vi "Get Cluster Info of Variant.vi"(8 "error in (no error)":errorcluster, 11 "Cluster Variant":variant) -> (0 "error out":errorcluster, 1 "mem_size":i32, 2 "byte_alignment":i16, 3 "Cluster Info":T1[](array[typedef]), 4 "flattstring_size":u32)   [LabVIEW 2021, in "DataTypes_CIF_U.lvlib"]
uses:
  DataTypes_CIF_U.lvlib
  Typedef/Cluster Info.ctl
  <vilib>/Utility/Data Type/Type Definitions/Data Type.ctl
  Typedef/Errors.ctl
  Errors/Append Error Location.vi
  <vilib>/Utility/Data Type/NI_Data Type.lvlib
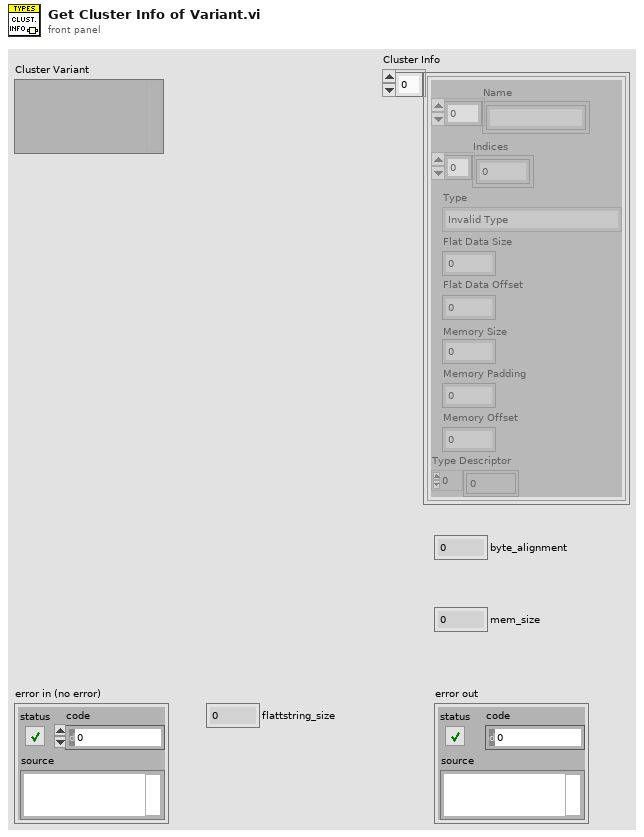
[diagram p1: front panel]
types:
  T1 = typedef "DataTypes_CIF_U.lvlib/Cluster Info.ctl" = cluster{"Name":string[], "Indices":i32[], "Type":T2, "Flat Data Size":u32, "Flat Data Offset":u32, "Memory Size":u32, "Memory Padding":u32, "Memory Offset":u32, "Type Descriptor":i16[]}
  T2 = typedef "NI_Data Type.lvlib/Data Type.ctl" = enum8{"Invalid Type", "Void", "I8", "I16", "I32", "I64", "U8", "U16", "U32", "U64", "Single Float", "Double Float", "Extended Float", "Single Complex", "Double Complex", "Extended Complex", "Enum U8", "Enum U16", "Enum U32", "Enum U64", "Single Float With Unit", "Double Float With Unit", "Extended Float With Unit", "Single Complex with Unit", "Double Complex with Unit", "Extended Complex with Unit", "Boolean", "String", "Path", "Picture", "Tag", "Array", "Cluster", "Variant", "LV Variant", "Waveform", "Timestamp", "Digital Waveform", "Digital Data", "ExpressData", "Refnum", "External Data", "VI", "Poly VI", "LabVIEW Class Instance", "Fixed Point", "Set Collection", "Map Collection"}
  T3 = typedef "DataTypes_CIF_U.lvlib/Errors.ctl" = enum16{"Too few bytes", "Unsupported Type"}
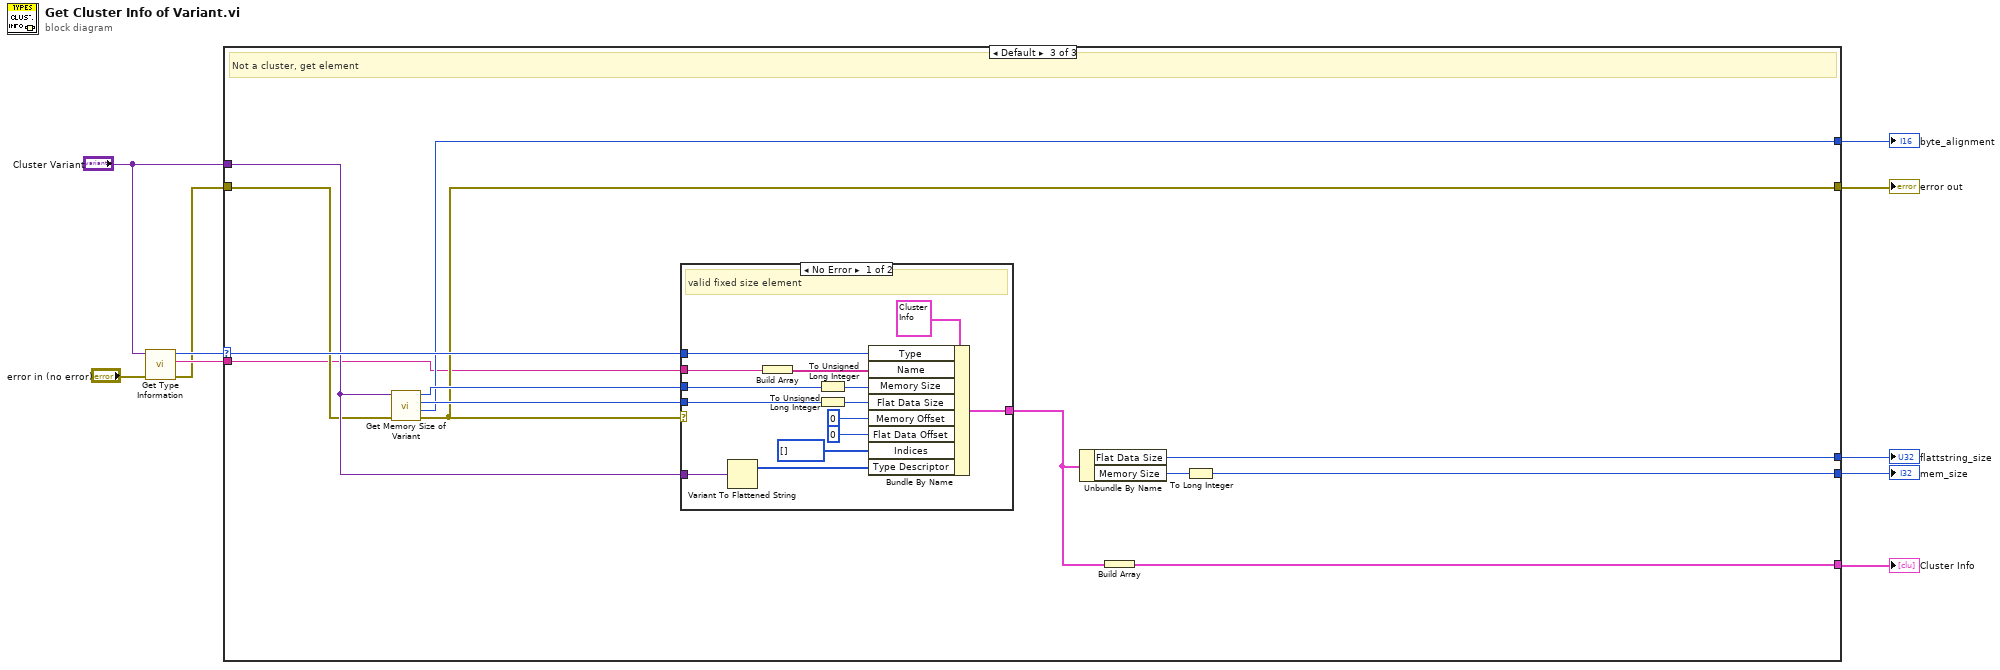
[diagram p0: block diagram]
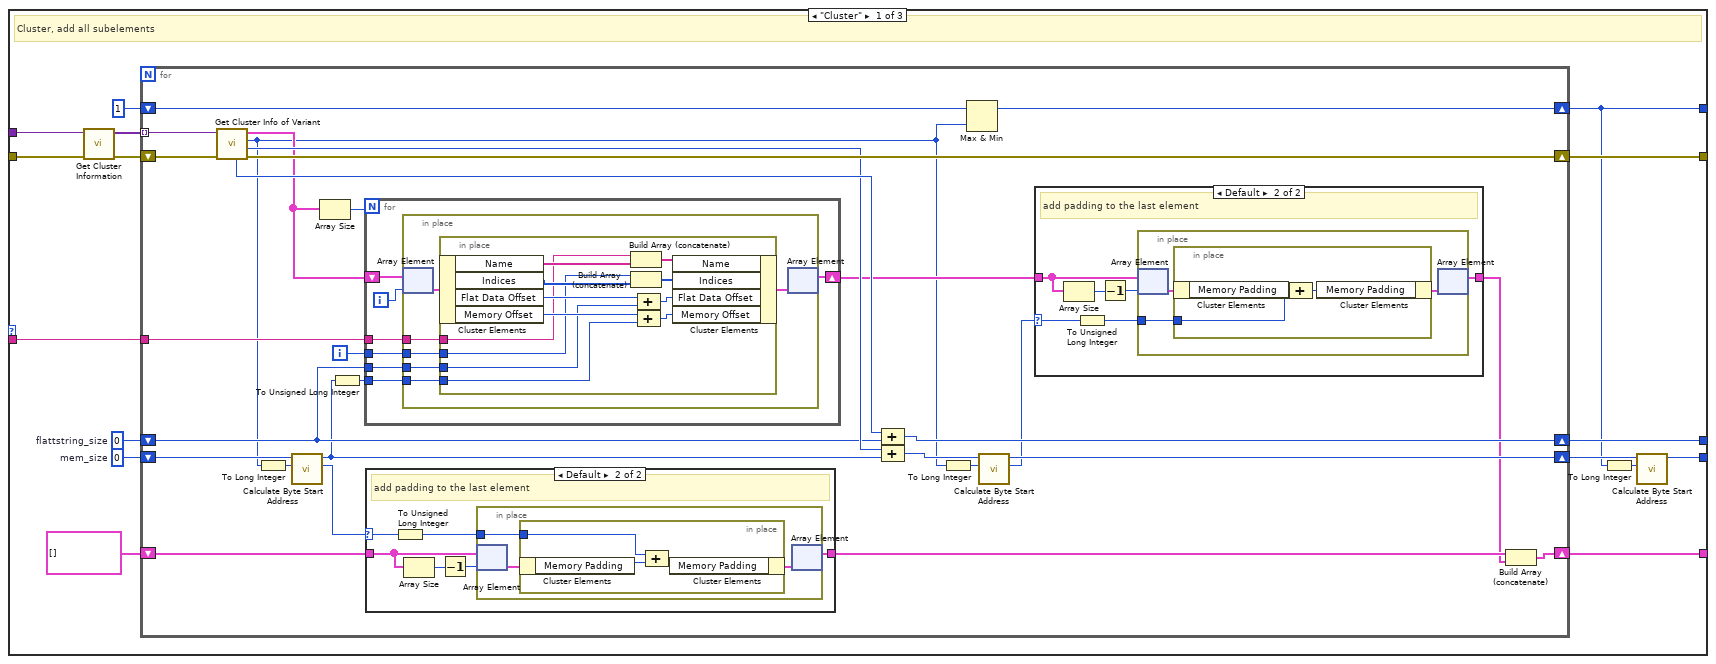
[diagram p2: hidden frame]
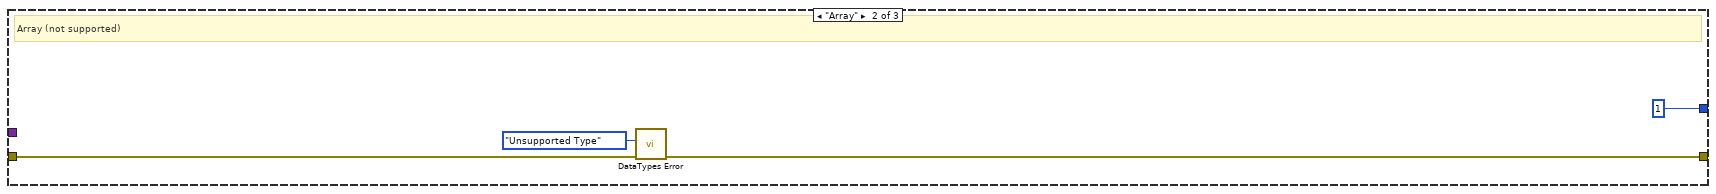
[diagram p5: hidden frame]
diagram:
  n1 = call <vilib>:"Get Type Information.vi"("error in (no error)"="error in (no error)", "variant"="Cluster Variant") -> ("error out"=w1:errorcluster, "name"=w6:string, "type"=w10:T2)  [unwired: 5 in, 2 out]
  n2 = case shown="Default" w10 {
    selector: w10 -> [_ _ w122]
    tunnel: w6 -> [w21 _ w113]
    tunnel: [w17 _ w111] -> w5
    tunnel: "Cluster Variant" -> [w26 _ w121]
    tunnel: w1 -> [w25 w108 w120]
    tunnel: [w23 w106 w115] -> w8
    tunnel: [w11 i16 1 ("byte_alignment") w114] -> w7
    tunnel: [w16 _ w117] -> w4
    tunnel: [w14 _ w112] -> w3
    frame "Cluster" {
      w20 = u32 0  # flattstring_size
      w19 = 0  # mem_size
      # "Cluster, add all subelements"
      n3 = call <vilib>:"Get Cluster Information.vi"("error in (no error)"=w25, "variant"=w26) -> ("error out"=w24:errorcluster, "cluster elements"=w18:variant[])  [unwired: 8 in]
      n4 = for {
        tunnel: w18 -> [w54] mode=indexing
        shift-right: [w52] -> w23
        shift-left: w24 -> [w53]
        shift-right: [w36] -> w11
        shift-left: i16 1 ("byte_alignment") -> [w51]
        tunnel: w21 -> [w49]
        shift-right: [w46] -> w16
        shift-left: w20 -> [w41]
        shift-right: [w45] -> w15
        shift-left: w19 -> [w48]
        shift-right: [w47] -> w17
        shift-left: T1[] [] -> [w38]
        i -> [w50]
        n5 = call "Get Cluster Info of Variant.vi"("error in (no error)"=w53, "Cluster Variant"=w54) -> ("error out"=w52:errorcluster, "mem_size"=w43:i32, "byte_alignment"=w27:i16, "Cluster Info"=w31:T1[], "flattstring_size"=w44:u32)  [unwired: 5 in]
        n6 = To Long Integer(number=w27) -> (32bit integer=w29:i32)
        n7 = call "Calculate Byte Start Address.vi"("data_byte_alignment"=w29, "byte_address_start"=w48) -> ("bytes_padding"=w39:i32, "byte_address_data"=w40:i32)  [unwired: 7 in]
        n8 = Array Size(array=w31) -> (size(s)=w32:i32)
        n9 = To Unsigned Long Integer(number=w40) -> (unsigned 32bit integer=w30:u32)
        n10 = for {
          N: w32 -> [_]
          tunnel: w50 -> [w87]
          tunnel: w49 -> [w86]
          shift-right: [w84] -> w35
          shift-left: w31 -> [w85]
          tunnel: w41 -> [w82]
          tunnel: w30 -> [w81]
          i -> [w83]
          n11 = in-place {
            in-place-border: w87 -> [w93]
            in-place-border: w86 -> [w92]
            in-place-border: w82 -> [w89]
            in-place-border: w81 -> [w88]
            n12 = in-place-array #1(w85, w83) -> (w91:T1)
            n13 = in-place {
              in-place-border: w92 -> [w97]
              in-place-border: w93 -> [w96]
              in-place-border: w88 -> [w94]
              in-place-border: w89 -> [w95]
              n14 = in-place-cluster #2(w91) -> ("Name"=w105:string[], "Indices"=w102:i32[], "Flat Data Offset"=w99:u32, "Memory Offset"=w101:u32)
              n15 = Build Array (concatenate)(w97, w105) -> (w104:string[])
              n16 = Build Array (concatenate)(w96, w102) -> (w103:i32[])
              n17 = Compound Arithmetic op=ADD(w99, w95) -> (w98:u32)
              n18 = Compound Arithmetic op=ADD(w101, w94) -> (w100:u32)
              n19 = in-place-cluster #2("Name"=w104, "Indices"=w103, "Flat Data Offset"=w98, "Memory Offset"=w100) -> (w90:T1)
            }
            n20 = in-place-array #1(w90) -> (w84:T1[])  [unwired: 1 out]
          }
        }
        n21 = case shown="Default" w39 {
          selector: w39 -> [_ w71]
          tunnel: w38 -> [w68 w74]
          tunnel: [w68 w70] -> w37
          frame 0 {
          }
          frame Default {
            # "add padding to the last element"
            n22 = To Unsigned Long Integer(number=w71) -> (unsigned 32bit integer=w69:u32)
            n23 = Array Size(array=w74) -> (size(s)=w72:i32)
            n24 = Decrement(x=w72) -> (x-1=w73:i32)
            n25 = in-place {
              in-place-border: w69 -> [w75]
              n26 = in-place-array #3(w74, w73) -> (w77:T1)
              n27 = in-place {
                in-place-border: w75 -> [w79]
                n28 = in-place-cluster #4(w77) -> ("Memory Padding"=w80:u32)
                n29 = Compound Arithmetic op=ADD(w79, w80) -> (w78:u32)
                n30 = in-place-cluster #4("Memory Padding"=w78) -> (w76:T1)
              }
              n31 = in-place-array #3(w76) -> (w70:T1[])  [unwired: 1 out]
            }
          }
        }
        n32 = Compound Arithmetic op=ADD(w44, w41) -> (w46:u32)
        n33 = Compound Arithmetic op=ADD(w43, w40) -> (w42:i32)
        n34 = To Long Integer(number=w27) -> (32bit integer=w28:i32)
        n35 = Max & Min(x=w51, y=w27) -> (max(x,y)=w36:i16)  [unwired: 1 out]
        n36 = call "Calculate Byte Start Address.vi"("data_byte_alignment"=w28, "byte_address_start"=w42) -> ("bytes_padding"=w33:i32, "byte_address_data"=w45:i32)  [unwired: 7 in]
        n37 = case shown="Default" w33 {
          selector: w33 -> [_ w58]
          tunnel: w35 -> [w55 w61]
          tunnel: [w55 w57] -> w34
          frame 0 {
          }
          frame Default {
            # "add padding to the last element"
            n38 = Array Size(array=w61) -> (size(s)=w59:i32)
            n39 = To Unsigned Long Integer(number=w58) -> (unsigned 32bit integer=w56:u32)
            n40 = Decrement(x=w59) -> (x-1=w60:i32)
            n41 = in-place {
              in-place-border: w56 -> [w62]
              n42 = in-place-array #5(w61, w60) -> (w64:T1)
              n43 = in-place {
                in-place-border: w62 -> [w65]
                n44 = in-place-cluster #6(w64) -> ("Memory Padding"=w66:u32)
                n45 = Compound Arithmetic op=ADD(w66, w65) -> (w67:u32)
                n46 = in-place-cluster #6("Memory Padding"=w67) -> (w63:T1)
              }
              n47 = in-place-array #5(w63) -> (w57:T1[])  [unwired: 1 out]
            }
          }
        }
        n48 = Build Array (concatenate)(w37, w34) -> (w47:T1[])
      }
      n49 = To Long Integer(number=w11) -> (32bit integer=w12:i32)
      n50 = call "Calculate Byte Start Address.vi"("data_byte_alignment"=w12, "byte_address_start"=w15) -> ("byte_address_data"=w14:i32)  [unwired: 7 in, 1 out]
    }
    frame "Array" {
      # "Array (not supported)"
      n51 = call "DataTypes Error.vi"("error in (no error)"=w108, "Error"=Errors."Unsupported Type") -> ("error out"=w106:errorcluster)  [unwired: 9 in]
    }
    frame Default {
      # "Not a cluster, get element"
      n52 = call "Get Memory Size of Variant.vi"("error in (no error)"=w120, "data"=w121) -> ("error out"=w115:errorcluster, "byte_alignment"=w114:i16, "flatten_string_size"=w118:i32, "mem_size"=w119:i64)  [unwired: 6 in]
      n53 = case shown="No Error" w115 {
        tunnel: w113 -> [w131 _]
        tunnel: w121 -> [w136 _]
        tunnel: w122 -> [w123 _]
        tunnel: w119 -> [w134 _]
        tunnel: w118 -> [w133 _]
        tunnel: [w128 _] -> w110
        frame No Error {
          # "valid fixed size element"
          n54 = Variant To Flattened String(Variant=w136) -> (1:w124:i16[])  [unwired: 1 out]
          n55 = Build Array(w131) -> (w132:string[])
          n56 = To Unsigned Long Integer(number=w134) -> (unsigned 32bit integer=w127:u32)
          n57 = To Unsigned Long Integer(number=w133) -> (unsigned 32bit integer=w126:u32)
          n58 = Bundle By Name(cluster=T1 {"Name"=[], "Indices"=[], "Type"=enum."Invalid Type", "Flat Data Size"=0, "Flat Data Offset"=0, "Memory Size"=0, "Memory Padding"=0, "Memory Offset"=0, "Type Descriptor"=[]} ("output cluster"), "Type"=w123, "Name"=w132, "Memory Size"=w127, "Flat Data Size"=w126, "Memory Offset"=u32 0 ("mem_offs"), "Flat Data Offset"=u32 0 ("flattstring_offs"), "Indices"=i32[] [], "Type Descriptor"=w124) -> (w128:T1)
        }
        frame Error {
        }
      }
      n59 = Unbundle By Name(w110) -> ("Flat Data Size"=w117:u32, "Memory Size"=w116:u32)
      n60 = Build Array(w110) -> (w111:T1[])
      n61 = To Long Integer(number=w116) -> (32bit integer=w112:i32)
    }
  }
  "Cluster Info" <- w5
  "error out" <- w8
  "byte_alignment" <- w7
  "flattstring_size" <- w4
  "mem_size" <- w3
